vi "Sea-Level SWI Get Stimulus.vi"(7 "Sea-Level SWI":T2, 8 "error in (no error)":errorcluster, 11 "Handle":i32) -> (0 "error out":errorcluster, 3 "Handle":i32, 5 "SWI Position":T1)   [LabVIEW 2011]
uses:
  TypeDefs/Sea-Level SWI Position.ctl
  TypeDefs/Sea-Level SWI Adapter Info.ctl
  TypeDefs/Sea-Level SWI Access Mode.ctl
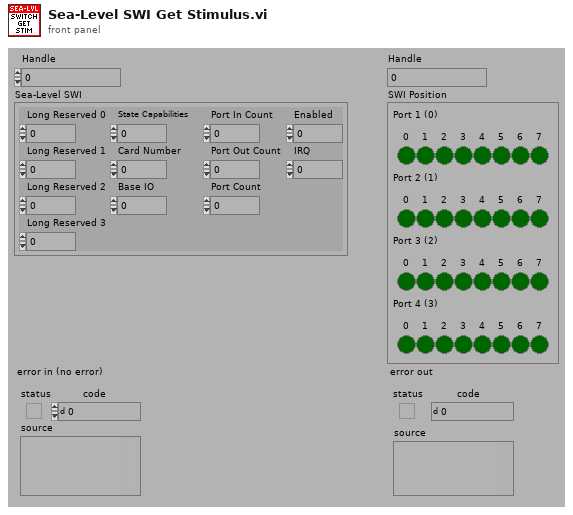
[diagram p1: front panel]
types:
  T1 = typedef "Sea-Level SWI Position.ctl" = cluster{"Port 1 (0)":cluster{"0":bool, "1":bool, "2":bool, "3":bool, "4":bool, "5":bool, "6":bool, "7":bool}, "Port 2 (1)":cluster{"0":bool, "1":bool, "2":bool, "3":bool, "4":bool, "5":bool, "6":bool, "7":bool}, "Port 3 (2)":cluster{"0":bool, "1":bool, "2":bool, "3":bool, "4":bool, "5":bool, "6":bool, "7":bool}, "Port 4 (3)":cluster{"0":bool, "1":bool, "2":bool, "3":bool, "4":bool, "5":bool, "6":bool, "7":bool}}
  T2 = typedef "Sea-Level SWI Adapter Info.ctl" = cluster{"Long Reserved 0":i32, "Long Reserved 1":i32, "Long Reserved 2":i32, "Long Reserved 3":i32, "State Capabilities":i32, "Card Number":i16, "Base IO":i16, "Port In Count":i8, "Port Out Count":i8, "Port Count":i8, "Enabled":i8, "IRQ":i16}
  T3 = typedef "Sea-Level SWI Access Mode.ctl" = enum16{"Relative", "Absolute"}
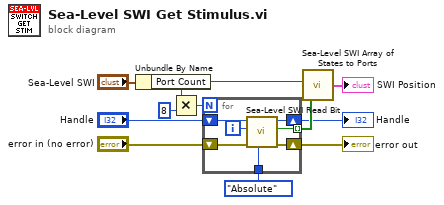
[diagram p0: block diagram]
diagram:
  n1 = Unbundle By Name("Sea-Level SWI") -> ("Port Count"=w1:i8)
  n2 = Multiply(x=w1, y=u32 8) -> (x*y=w8:u32)
  n3 = for {
    N: w8 -> [_]
    tunnel: [w13] -> w9 mode=indexing
    tunnel: Sea-Level_SWI_Access_Mode."Absolute" ("Access Mode (Relative)") -> [w12]
    shift-right: [w15] -> w5
    shift-left: "error in (no error)" -> [w18]
    shift-right: [w16] -> w4
    shift-left: "Handle" -> [w17]
    i -> [w14]
    n4 = call "Sea-Level SWI Read Bit.vi"("Access Mode (Relative)"=w12, "error in (no error)"=w18, "Bit Number"=w14, "Handle"=w17) -> ("error out"=w15:errorcluster, "State"=w13:bool, "Handle Out"=w16:i32)  [unwired: 1 in, 4 out]
  }
  "error out" <- w5
  "Handle" <- w4
  n5 = call "Sea-Level SWI Array of States to Ports.vi"("State Array"=w9, "Number of Ports"=w1) -> ("SWI Position"=→"SWI Position":T1)  [unwired: 2 out]
